vi "Pack and unpack DRAM data.vi"(2 "Write DRAM enable?":bool) -> (7 "Write DRAM done?":bool)   [LabVIEW 2015]
uses:
  <vilib>/Platform/TimedLoop/XDataNode/timing_clust.ctl
  <vilib>/Platform/TimedLoop/XDataNode/nitl_modes.ctl
  <vilib>/Platform/TimedLoop/XDataNode/wakeup.ctl
  OpenScan Labview code_20170126/DRAM data index.ctl
  <vilib>/rvi/Emulation/niFpgaSctlEmulationGetInTimedLoop.vi
  <vilib>/rvi/Emulation/niFpgaEmulationReportErrorSimple.vi
  <vilib>/rvi/Emulation/niFpgaGetClockAttributes.vi
  <vilib>/rvi/Emulation/niFpgaCriticalErrorInLSC.vi
  <vilib>/rvi/DataTransferAndStorage/Container/Common/niFpgaContainerGetUniqueNameForEmu.vi
  <vilib>/rvi/interface/RandomDataEmulation/niFpgaRandomDataHandleErrors.vi
  <vilib>/rvi/Memory/Memory_Emulation/niFpgaMemoryFastEmulationDramWriteAndRequestData.vi
  <vilib>/rvi/Memory/Memory_Emulation/niFpgaMemoryEmulationDramWriteAndRequestData.vi
  <vilib>/rvi/Memory/Memory_Emulation/niFpgaMemoryEmulationDramWriteAndRequestDataApplyByteEnables.vi
  <vilib>/rvi/Emulation/niFpgaProcessEmulError.vi
  <vilib>/Platform/TimedLoop/XDataNode/XDataNode.xnode
  <vilib>/rvi/DataTransferAndStorage/Container/XNode/niFpgaContainer.xnode
  <vilib>/rvi/Memory/Memory_Emulation/niFpgaMemoryEmulationDramRetrieveData.vi
  <vilib>/rvi/interface/RandomDataEmulation/nirviRandomDataFpgaReadWriteTemplate.vi
  <vilib>/Platform/TimedLoop/XDataNode/XDNodeRunTimeDep.lvlib
panel:
  in  "Byte Enables":i64
  out "Data":T1
  out "packed data":T1
  out "Read DRAM begin?":bool=TRUE
  out "Write DRAm begin?":bool=TRUE
  out "unpacked data readed":i32
  out "Read DRAM address":u32
  out "Write DRAM address":u32
  in  "Total elements to write":i32
  out "read DRAM done?":bool
  in  "Total packed data to write?":u32
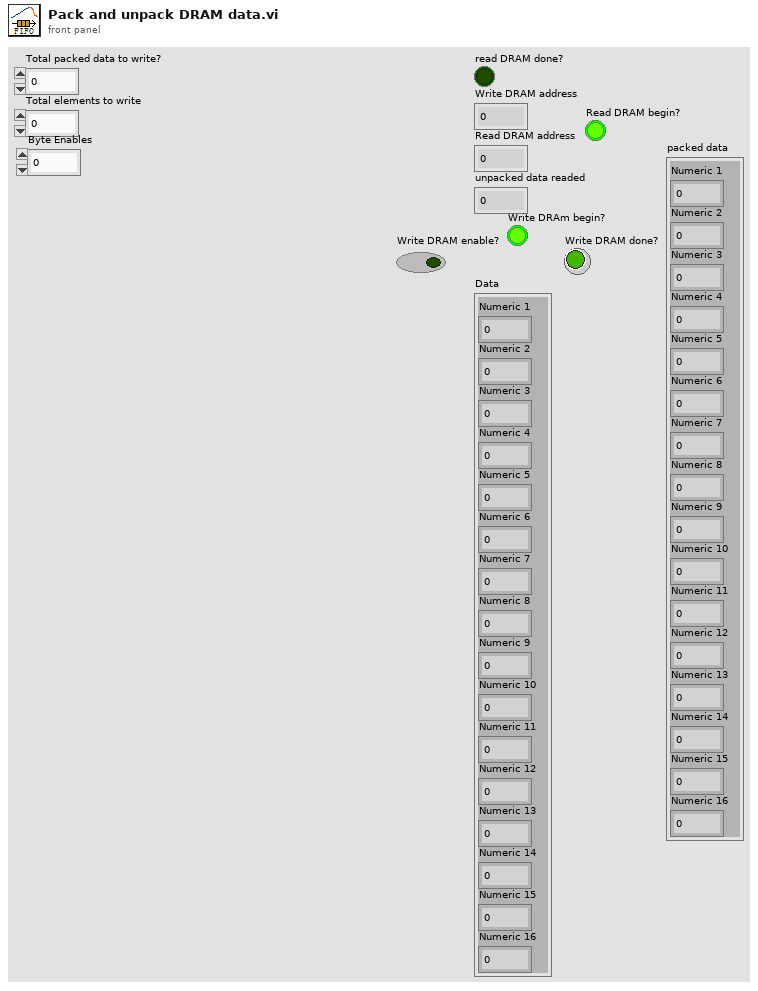
[diagram p1: front panel]
types:
  T1 = cluster{"Numeric 1":u32, "Numeric 2":u32, "Numeric 3":u32, "Numeric 4":u32, "Numeric 5":u32, "Numeric 6":u32, "Numeric 7":u32, "Numeric 8":u32, "Numeric 9":u32, "Numeric 10":u32, "Numeric 11":u32, "Numeric 12":u32, "Numeric 13":u32, "Numeric 14":u32, "Numeric 15":u32, "Numeric 16":u32}
  T2 = typedef "DRAM data index.ctl" = enum16{"Numeric 1", "Numeric 2", "Numeric 3", "Numeric 4", "Numeric 5", "Numeric 6", "Numeric 7", "Numeric 8", "Numeric 9", "Numeric 10", "Numeric 11", "Numeric 12", "Numeric 13", "Numeric 14", "Numeric 15", "Numeric 16"}
  T3 = enum16{"Wait on Trigger", "Write DRAM", "Read DRAM"}
  T4 = typedef "XDNodeRunTimeDep.lvlib/timing_clust.ctl" = cluster{"Expected End [f-1]":u64, "Actual End [f-1]":u64, "Finished Late? [f-1]":bool, "Expected End [i-1]":u64, "Actual End [i-1]":u64, "Finished Late? [i-1]":bool, "Expected Start [i]":u64, "Actual Start [i]":u64, "Expected Start [f]":u64, "Actual Start [f]":u64, "Source Name":string, "Structure Name":string, "Period":i64, "Deadline":i64, "Offset":i64, "Start":i64, "Priority":i32, "Timeout":i32, "Mode":T5, "Wakeup Reason":T6, "Error":errorcluster, "Source Type":string, "Secondary Source Type":string, "Global End Time":u64, "Global Start Time":u64, "Frame Duration":u64, "Iteration Duration":u64, "Assigned CPU":i32, "I/O Scan Engine Mode":u32}
  T5 = typedef "XDNodeRunTimeDep.lvlib/nitl_modes.ctl" = enum32{"No Change", "Process missed periods, maintain original phase", "Discard missed periods, maintain original phase", "Process missed periods, ignore original phase", "Discard missed periods, ignore original phase"}
  T6 = typedef "XDNodeRunTimeDep.lvlib/wakeup.ctl" = enum32{"Normal", "Aborted", "Asynchronous wakeup", "Timing source error", "Timed loop error", "Timeout"}
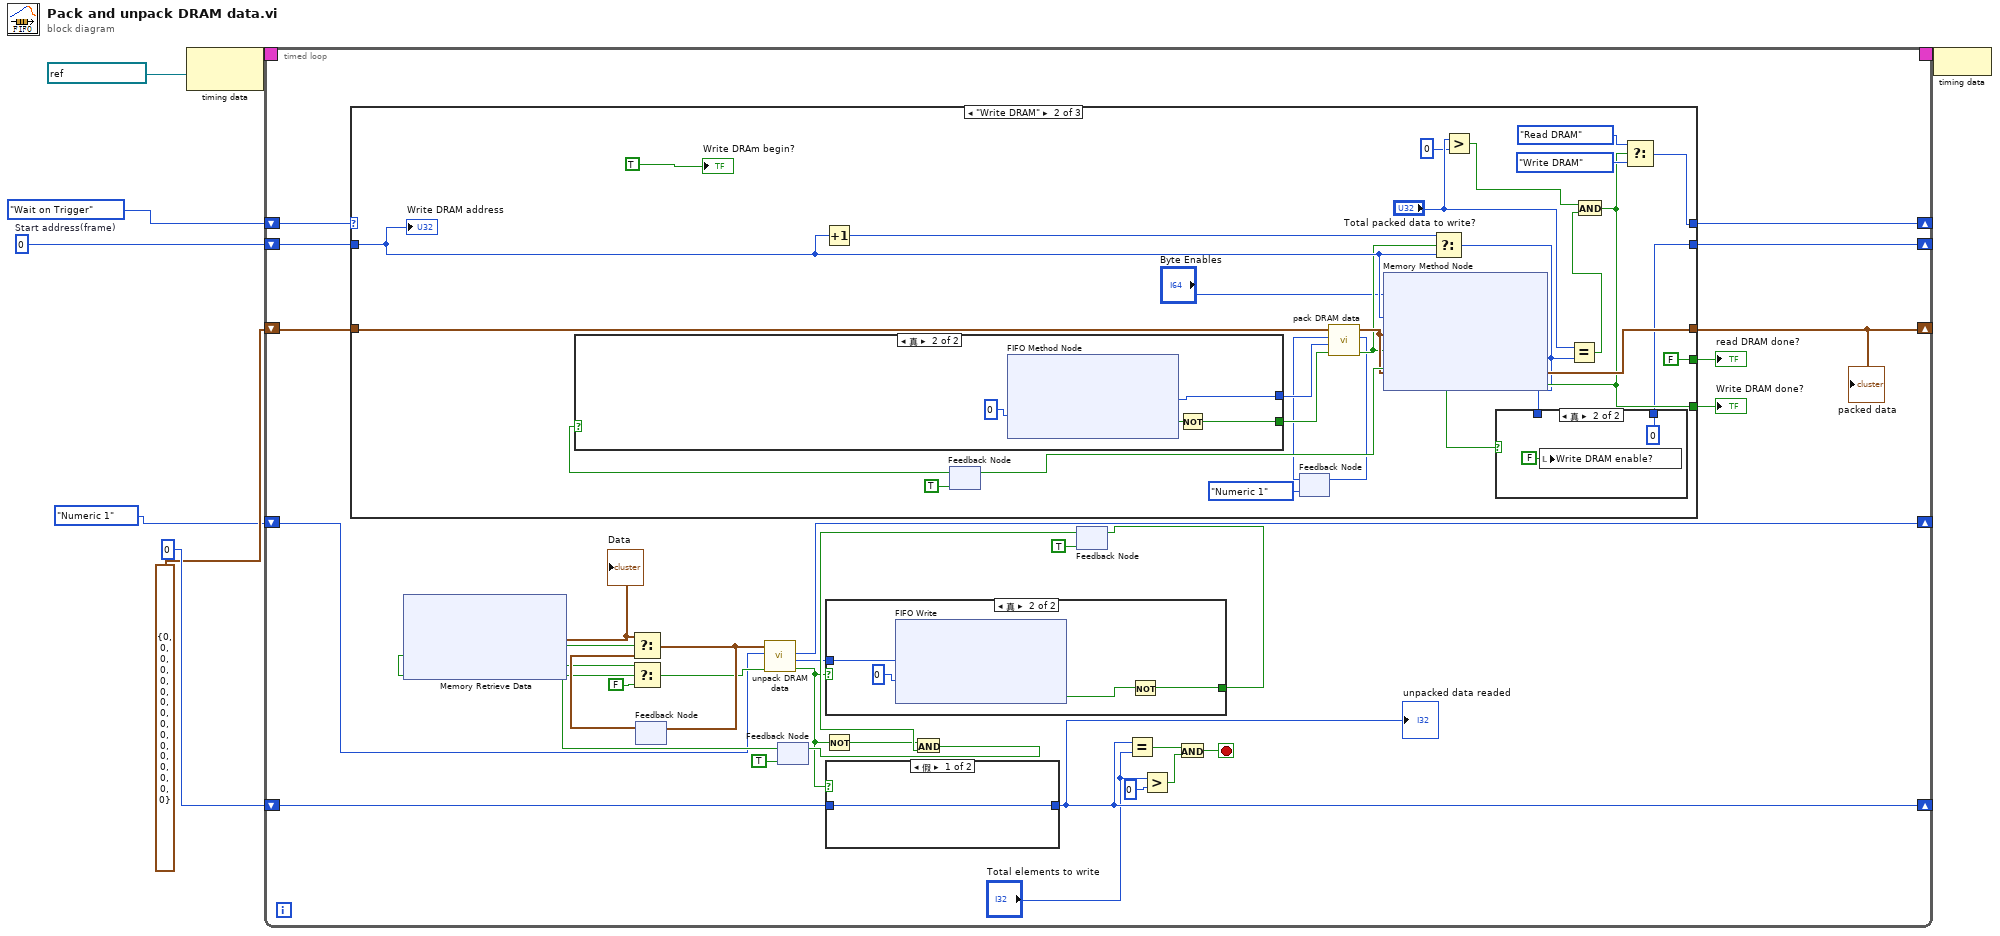
[diagram p0: block diagram]
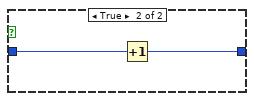
[diagram p2: hidden frame]
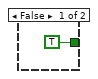
[diagram p3: hidden frame]
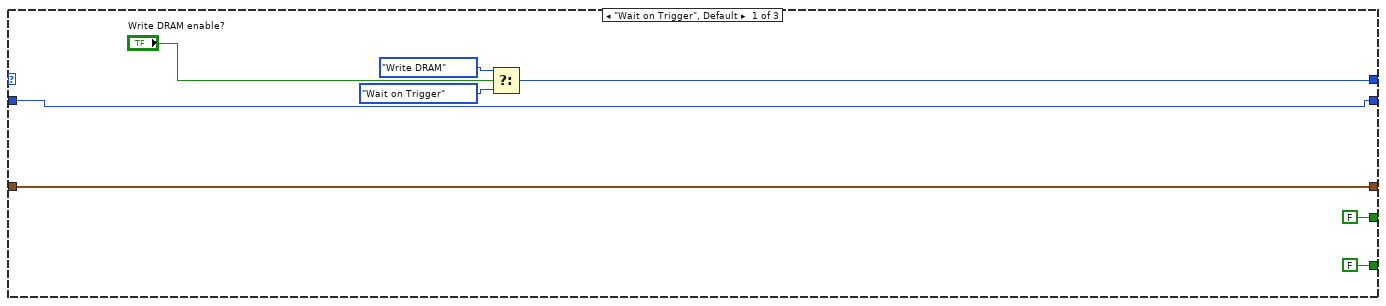
[diagram p4: hidden frame]
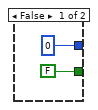
[diagram p6: hidden frame]
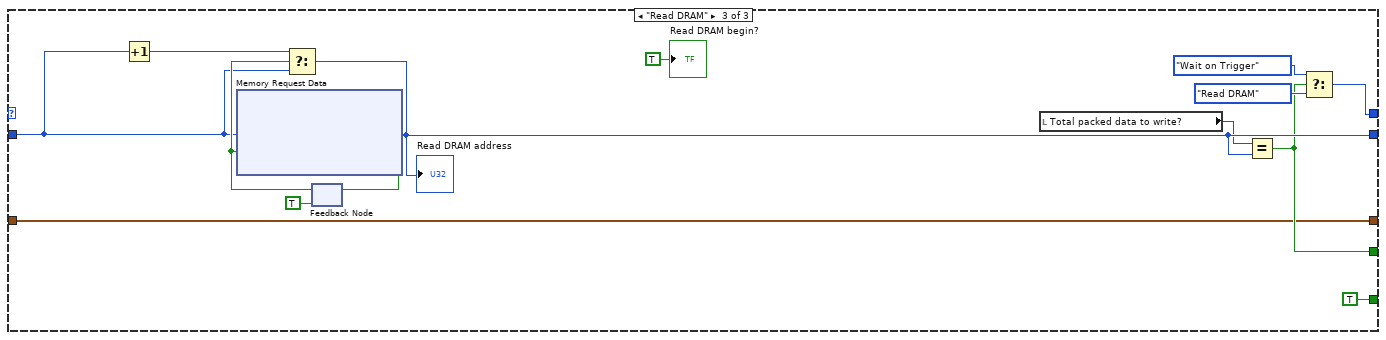
[diagram p7: hidden frame]
diagram:
  w6 = u32 0  # Start address(frame)
  n1 = node-c288(refnum<k21> "DRAM Clock" ("Source Name")) -> (w8:T4)
  n2 = timed-loop {
    timing: w8 -> [_]
    timing-out: [_] -> w7
    shift-right: [w39] -> _
    shift-left: T3."Wait on Trigger" -> [w37]
    shift-right: [w38] -> _
    shift-left: w6 -> [w40]
    shift-right: [w24] -> _
    shift-left: 0 ("Timeout") -> [w25]
    shift-right: [w15] -> _
    shift-left: T1 {"Numeric 1"=0, "Numeric 2"=0, "Numeric 3"=0, "Numeric 4"=0, "Numeric 5"=0, "Numeric 6"=0, "Numeric 7"=0, "Numeric 8"=0, "Numeric 9"=0, "Numeric 10"=0, "Numeric 11"=0, "Numeric 12"=0, "Numeric 13"=0, "Numeric 14"=0, "Numeric 15"=0, "Numeric 16"=0} ("packer in") -> [w16]
    shift-right: [w13] -> _
    shift-left: DRAM_data_index."Numeric 1" ("DRAM pack index in") -> [w9]
    stop <- w18 stop-if-true
    n3 = case shown="\"Write DRAM\"" w37 {
      tunnel: w40 -> [w55 w70 w100]
      tunnel: [w55 w57 w99] -> w38
      tunnel: [w56 w79 w95] -> w39
      tunnel: [FALSE w64 TRUE] -> w17
      tunnel: [FALSE FALSE w94] -> w30
      tunnel: w16 -> [w50 w72 w93]
      tunnel: [w50 w71 w93] -> w15
      frame "Wait on Trigger", Default {
        n4 = Select(t=T3."Write DRAM", s="Write DRAM enable?", f=T3."Wait on Trigger") -> (s? t:f=w56:T3)
      }
      frame "Write DRAM" {
        n5 = Increment(x=w70) -> (x+1=w80:u32)
        n6 = feedback #1(TRUE ("Ready for Input")) -> (w81:bool)
        n7 = case shown="真" w81 {
          tunnel: [FALSE w89] -> w74
          tunnel: [u32 0 ("Element") w88] -> w73
          frame False {
          }
          frame True {
            n8 = xnode ("FIFO Method Node")("超时"=0 ("Timeout")) -> ("元素"=w88:u32, "超时？"=w90:bool)  [unwired: 1 in, 1 out]
            n9 = Not(x=w90) -> (.not. x?=w89:bool)
          }
        }
        n10 = feedback #2(DRAM_data_index."Numeric 1" ("Galvo index out")) -> (w61:T2)
        n11 = call "pack DRAM data.vi"("input valid?"=w74, "data to be packed"=w73, "DRAM Index in"=w61, "packer in"=w72) -> ("output valid?"=w69:bool, "DRAM Index out"=w62:T2, "packer out"=w71:T1)  [unwired: 5 in]
        n12 = feedback-in #2(w62) -> ()
        n13 = xnode ("Memory Method Node")("地址"=w70, "数据"=w71, "输入有效"=w69, "字节启用"="Byte Enables") -> ("输入就绪"=w82:bool)  [unwired: 1 in, 1 out]
        n14 = feedback-in #1(w82) -> ()
        n15 = Select(t=w80, s=w69, f=w70) -> (s? t:f=w58:u32)
        n16 = Greater?(x="Total packed data to write?", y=u32 0) -> (0:w66:bool)
        n17 = Equal?(x="Total packed data to write?", y=w58) -> (x = y?=w65:bool)
        n18 = And(x=w66, y=w65) -> (x .and. y?=w64:bool)
        n19 = case shown="真" w64 {
          tunnel: w58 -> [w83 _]
          tunnel: [w83 u32 0 ("Start address(frame)")] -> w57
          frame False {
          }
          frame True {
            n20 = local write "Write DRAM enable?"(FALSE ("Write DRAM enable?")) -> ()
          }
        }
        n21 = Select(t=T3."Read DRAM", s=w64, f=T3."Write DRAM") -> (s? t:f=w79:T3)
        "Write DRAM address" <- w70
        "Write DRAm begin?" <- TRUE
      }
      frame "Read DRAM" {
        n22 = Increment(x=w100) -> (x+1=w101:u32)
        n23 = feedback #3(TRUE ("Ready for Input")) -> (w102:bool)
        n24 = xnode ("Memory Request Data")("地址"=w100, "输入有效"=w102) -> ("输入就绪"=w104:bool)  [unwired: 1 in, 1 out]
        n25 = Select(t=w101, s=w102, f=w100) -> (s? t:f=w99:u32)
        "Read DRAM address" <- w99
        n26 = feedback-in #3(w104) -> ()
        n27 = local read "Total packed data to write?"() -> (w98:u32)
        n28 = Equal?(x=w98, y=w99) -> (x = y?=w94:bool)
        n29 = Select(t=T3."Wait on Trigger", s=w94, f=T3."Read DRAM") -> (s? t:f=w95:T3)
        "Read DRAM begin?" <- TRUE
      }
    }
    "Write DRAM done?" <- w17
    "read DRAM done?" <- w30
    "packed data" <- w15
    n30 = feedback #4() -> (w33:T1)  [unwired: 1 in]
    n31 = feedback #5(TRUE) -> (w26:bool)
    n32 = xnode ("Memory Retrieve Data")("输出就绪"=w26) -> ("数据"=w34:T1, "输出有效"=w32:bool)  [unwired: 1 in, 1 out]
    "Data" <- w34
    n33 = Select(t=w34, s=w32, f=w33) -> (s? t:f=w14:T1)
    n34 = Select(t=w32, s=w26, f=FALSE) -> (s? t:f=w12:bool)
    n35 = feedback-in #4(w14) -> ()
    n36 = call "unpack DRAM data.vi"("input valid?"=w12, "DRAM pack index in"=w9, "packer in"=w14) -> ("output valid?"=w10:bool, "Unpacked data"=w11:u32, "DRAM pack index out"=w13:T2)  [unwired: 5 in, 1 out]
    n37 = Not(x=w10) -> (.not. x?=w28:bool)
    n38 = case shown="真" w10 {
      tunnel: [TRUE w46] -> w36
      tunnel: w11 -> [_ w45]
      frame False {
      }
      frame True {
        n39 = xnode ("FIFO Write")("元素"=w45, "超时"=0 ("Timeout")) -> ("超时？"=w48:bool)  [unwired: 1 in, 1 out]
        n40 = Not(x=w48) -> (.not. x?=w46:bool)
      }
    }
    n41 = case shown="假" w10 {
      tunnel: w25 -> [w41 w43]
      tunnel: [w41 w42] -> w24
      frame False {
      }
      frame True {
        n42 = Increment(x=w43) -> (x+1=w42:i32)
      }
    }
    "unpacked data readed" <- w24
    n43 = feedback-in #6(w36) -> ()
    n44 = feedback #6(TRUE ("Timed Out?")) -> (w29:bool)
    n45 = And(x=w28, y=w29) -> (x .and. y?=w27:bool)
    n46 = feedback-in #5(w27) -> ()
    n47 = Equal?(x=w24, y="Total elements to write") -> (x = y?=w20:bool)
    n48 = Greater?(x="Total elements to write", y=0) -> (0:w19:bool)
    n49 = And(x=w20, y=w19) -> (x .and. y?=w18:bool)
  }
  n50 = node-c288(w7) -> ()
